vi "Analyze dIdV.vi"() -> ()   [LabVIEW 2021, in "dIdV State.lvclass"]
uses:
  dIdV State/dIdV State.lvclass
  Controls/PCS Config.ctl
  Parameters.ctl
  dIdV State/dIdV State.lvclass/dIdV State.ctl
  <vilib>/Utility/config.llb/NI_LVConfig.lvlib
  <vilib>/Utility/TDMS File Viewer/NI_TDMS File Viewer.lvlib
panel:
  in  "Array - String":string[](array[string])
  in  "Input onfiguration":T1={"File Path"=path "U:/My Documents/Projects/Eremets/NV/IV/Data/August_2022/080922/m008_080922.tdms", "from scan..."=0, "...to scan"=4, "Resistance in series"=25.65079365079365, "Correct conductance "=TRUE, "Model parameters"={"Delta"=0.025, "Gama"=0.0, "Z"=0.0, "P"=0.0, "T"=1.0, "Integration range"=2.0, "Resolution"=0.0001}, "Scale"=0.5473251028806585, "Offset"=0.0, "Other channels"=[]} {"Offset" scale=0.0..1.0; "Scale" scale=0.0..1.0; "Model parameters"."Resolution" format="%#_6peV"; "Model parameters"."Integration range" format="%#_6peV"; "Model parameters"."T" format="%#_6pK"; "Model parameters"."Delta" step=0.001 format="%#_6peV"; "Model parameters"."Gama" step=0.001 format="%#_6peV"; "Resistance in series" scale=75.0..85.0}
  in  "Tab Control":enum32{"Input", "Model", "Evaluations"}(tab)
  in  "View Button":bool
  out "Scans in file":i32
  out "All scans":cluster{dbl[], dbl[]}[](graph)
  in  "Open Button":bool
  out "Other values":string[](array[string])
  out "BTK model":cluster{dbl[], dbl[]}[](graph)
  out "V-I":cluster{"I":dbl[], dbl[]}[](graph)
  in  "Model Button":bool
  out "BSC Delta T":dbl=0.003040195174884819 format="%#_6peV"
  out "BSC Delta 0":dbl=0.003040195174884819 format="%#_6peV"
  in  "Physical quantities":T3={"Tc"=20.0, "T"=20.0, "Tc-> Delta factor"=1.764, "Hc2 at T"=20.0, "H"=20.0} {"H" format="%#_6pT"; "Hc2 at T" format="%#_6pT"; "Tc-> Delta factor" format="%#_6p"; "T" format="%#_6pK"; "Tc" format="%#_6pK"}
  out "BSC Delta T H":dbl=0.003040195174884819 format="%#_6peV"
  in  "Write cfg":bool
  in  "Read cfg":bool
  in  "Process Stop Button":bool
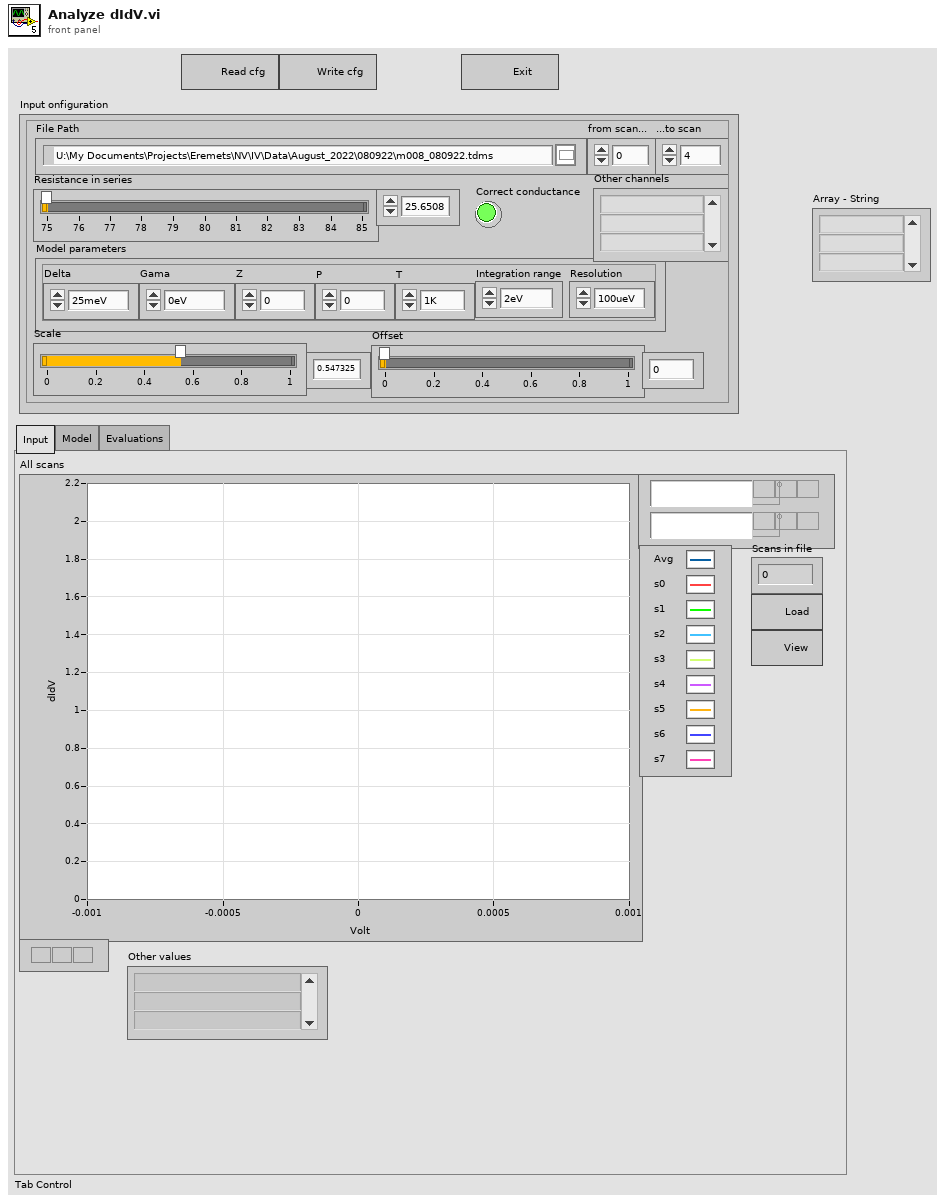
[diagram p1: front panel]
types:
  T1 = typedef "PCS Config.ctl" = cluster{"File Path":path, "from scan...":i32, "...to scan":i32, "Resistance in series":dbl, "Correct conductance ":bool, "Model parameters":T2, "Scale":dbl, "Offset":dbl, "Other channels":string[]}
  T2 = typedef "Parameters.ctl" = cluster{"Delta":dbl, "Gama":dbl, "Z":dbl, "P":dbl, "T":dbl, "Integration range":dbl, "Resolution":dbl}
  T3 = cluster{"Tc":dbl, "T":dbl, "Tc-> Delta factor":dbl, "Hc2 at T":dbl, "H":dbl}
  T4 = enum8{"Enabled", "Disabled", "Disabled and Grayed Out"}
  T5 = typedef "NI_LVConfig.lvlib/Config Data RefNum.ctl" = refnum<k1>
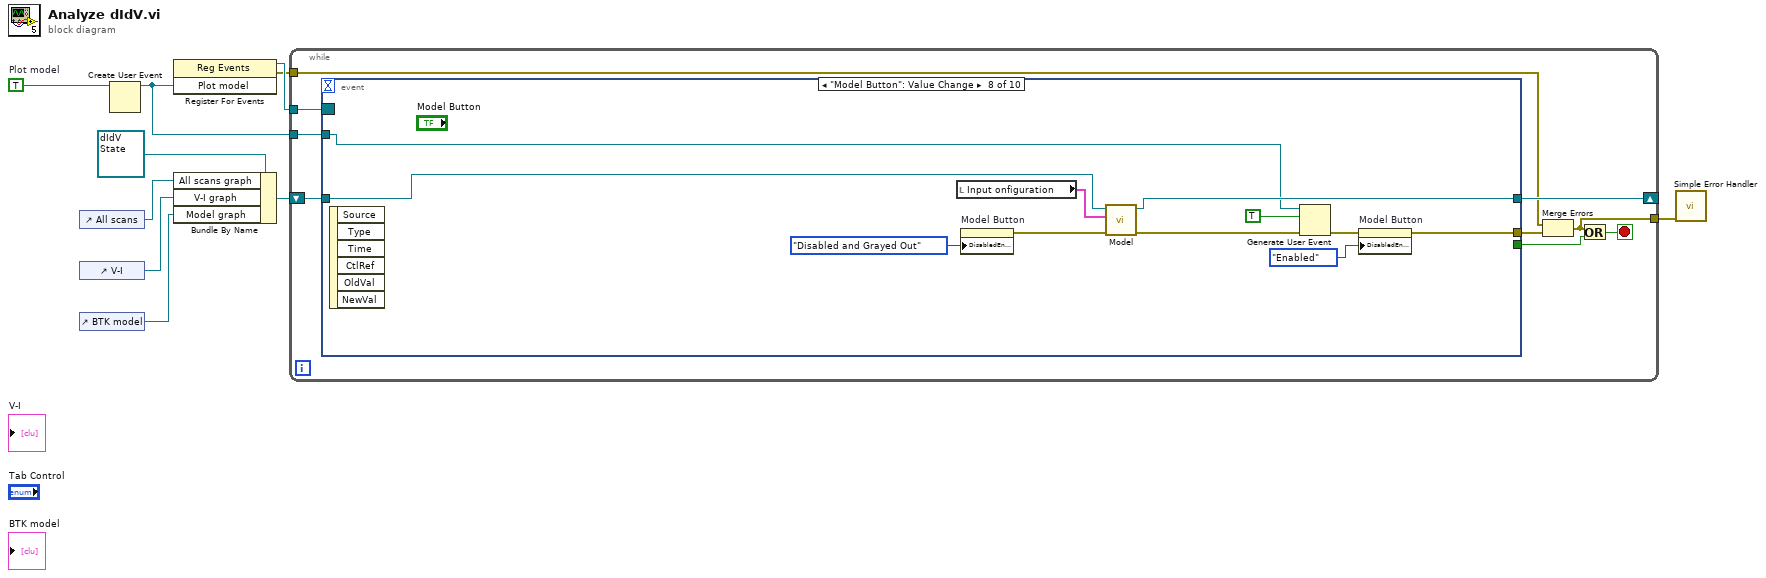
[diagram p0: block diagram]
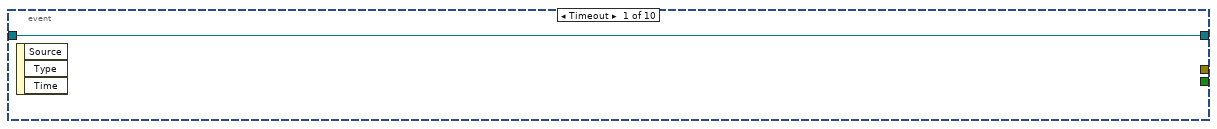
[diagram p2: hidden frame]
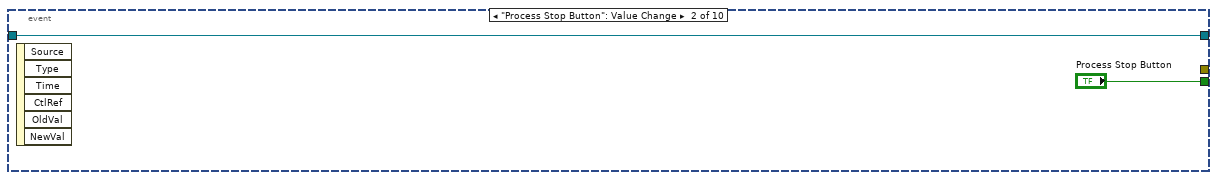
[diagram p3: hidden frame]
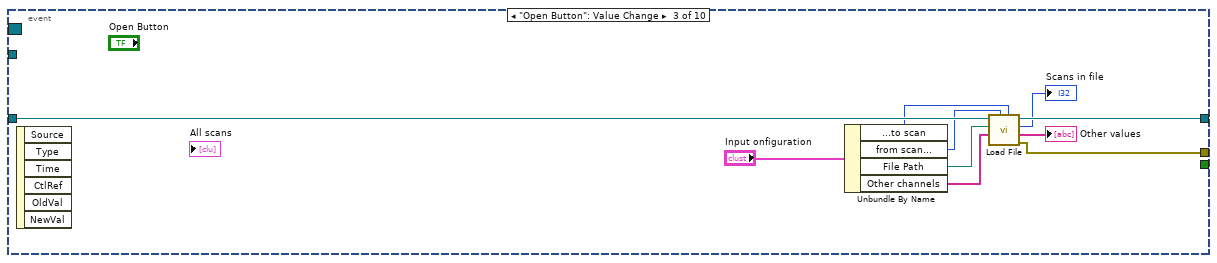
[diagram p4: hidden frame]
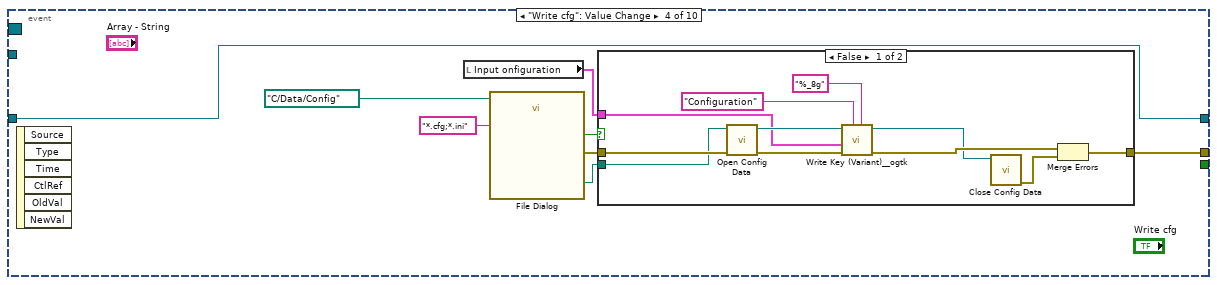
[diagram p5: hidden frame]
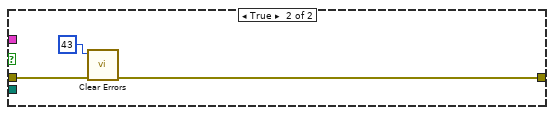
[diagram p6: hidden frame]
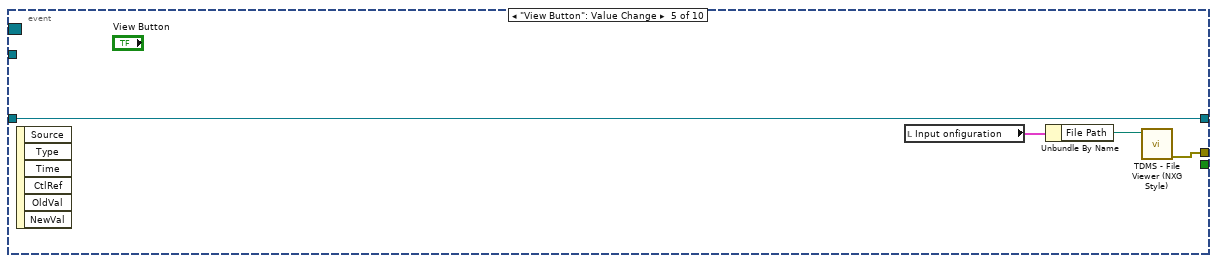
[diagram p7: hidden frame]
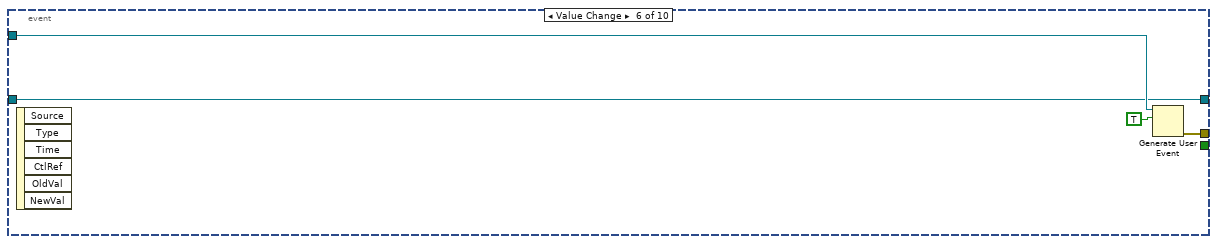
[diagram p8: hidden frame]
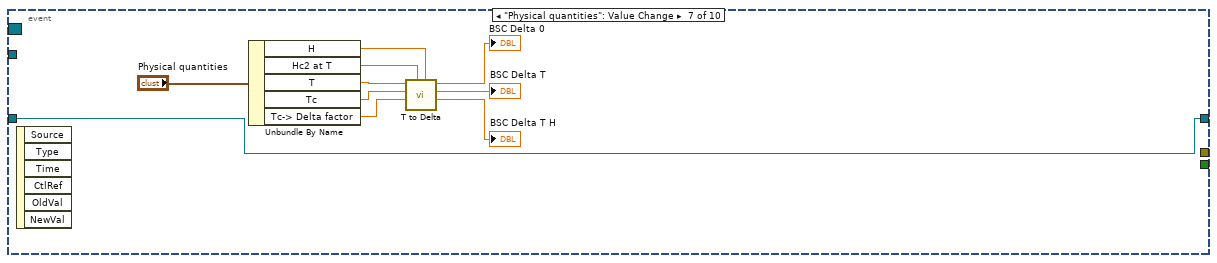
[diagram p9: hidden frame]
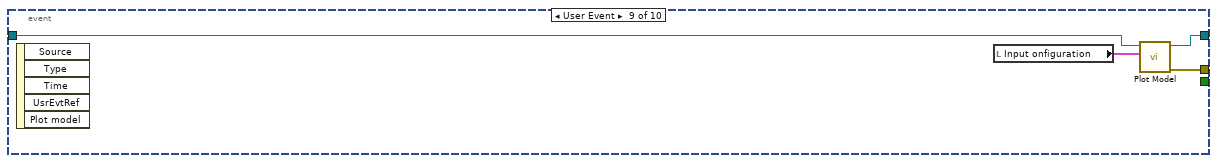
[diagram p10: hidden frame]
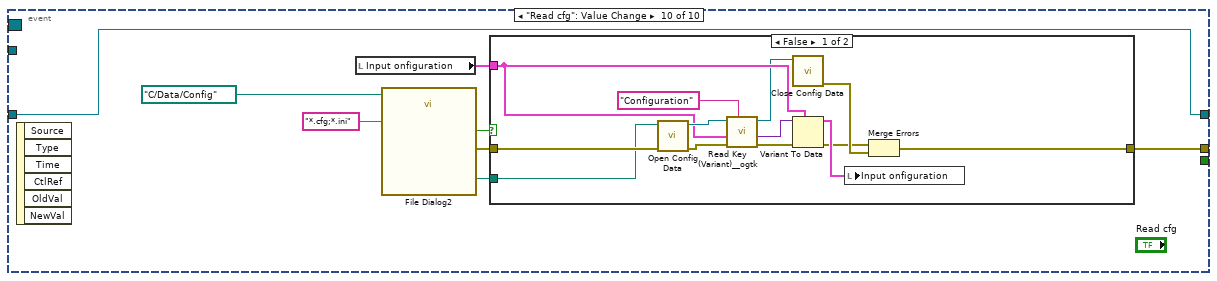
[diagram p11: hidden frame]
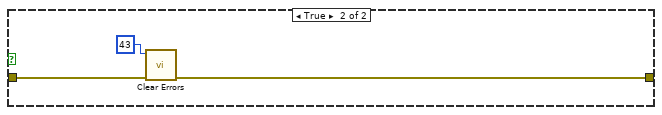
[diagram p12: hidden frame]
diagram:
  w4 = TRUE  # Plot model
  n1 = control-ref of="All scans"() -> (w8:refnum<vi>)
  n2 = control-ref of="V-I"() -> (w6:refnum<vi>)
  n3 = control-ref of="BTK model"() -> (w5:refnum<vi>)
  n4 = Create User Event(user event datatype=w4) -> (user event=w1:refnum<user-event>)  [unwired: 1 in, 1 out]
  n5 = register-events(w1) -> (reference out=w3:refnum<event-registration>, error out=w2:errorcluster)  [unwired: 2 in]
  n6 = Bundle By Name(cluster=refnum<class "dIdV State.lvclass"> refnum ("dIdV State.lvclass"), "All scans graph"=w8, "V-I graph"=w6, "Model graph"=w5) -> (w7:refnum<class "dIdV State.lvclass">)
  n7 = while {
    tunnel: [w13] -> w10
    shift-right: [w15] -> _
    shift-left: w7 -> [w16]
    tunnel: w3 -> [w14]
    tunnel: w2 -> [w12]
    tunnel: w1 -> [w11]
    stop <- w18 stop-if-true
    n8 = event shown="[7] \"Model Button\": Value Change" {
      selector: w14 -> [_ _ _ _ _ _ _ _ _ _]
      dyn-events: _ -> [_ _ _ _ _ _ _ _ _ _]
      timeout: _ -> [_ _ _ _ _ _ _ _ _ _]
      tunnel: [_ "Process Stop Button" _ _ _ _ _ _ _ _] -> w19
      tunnel: [_ _ w30 w36 w55 w61 _ w74 w85 w91] -> w17
      tunnel: w16 -> [w20 w21 w32 w35 w58 w59 w63 w83 w87 w90]
      tunnel: [w20 w21 w31 w35 w58 w59 w63 w82 w86 w90] -> w15
      tunnel: w11 -> [_ _ _ _ _ w62 _ w79 _ _]
      event Timeout {
        n9 = event-data() -> ()  [unwired: 1 in, 3 out]
      }
      event "Process Stop Button": Value Change {
        n10 = event-data() -> ()  [unwired: 1 in, 6 out]
      }
      event "Open Button": Value Change {
        n11 = event-data() -> ()  [unwired: 1 in, 6 out]
        n12 = Unbundle By Name("Input onfiguration") -> ("...to scan"=w27:i32, "from scan..."=w26:i32, "File Path"=w25:path, "Other channels"=w23:string[])
        n13 = call-dynamic "Load File.vi"("...to scan"=w27, "from scan..."=w26, "Other channels"=w23, "File Path"=w25, "dIdV State in"=w32) -> ("error out"=w30:errorcluster, "Other values"=→"Other values":string[], "Number of scans"=→"Scans in file":i32, "dIdV State out"=w31:refnum<class "dIdV State.lvclass">)  [unwired: 3 in]
      }
      event "Write cfg": Value Change {
        n14 = event-data() -> ()  [unwired: 1 in, 6 out]
        n15 = local read "Input onfiguration"() -> (w34:T1)
        n16 = call "File Dialog"("start path"=path "C:/Data/Config", "pattern (all files)"="*.cfg;*.ini") -> ("selected path"=w39:path, "cancelled"=w40:bool, "error out"=w37:errorcluster)  [unwired: 10 in, 1 out]
        n17 = case shown="False" w40 {
          tunnel: w39 -> [w44 _]
          tunnel: w37 -> [w45 w54]
          tunnel: [w42 w53] -> w36
          tunnel: w34 -> [w43 _]
          frame False {
            n18 = call <vilib>:"Open Config Data.vi"("error in (no error)"=w45, "configuration file path"=w44) -> ("error out"=w47:errorcluster, "refnum"=w46:T5)  [unwired: 7 in, 1 out]
            n19 = call <userlib>:"Write Key (Variant)__ogtk.vi"("float number format"="%_8g", "section"="Configuration", "error in (no error)"=w47, "key-value"=w43, "refnum"=w46) -> ("error out"=w49:errorcluster, "refnum out"=w48:T5)  [unwired: 5 in]
            n20 = call <vilib>:"Close Config Data.vi"("refnum"=w48) -> ("error out"=w50:errorcluster)  [unwired: 9 in, 1 out]
            n21 = Merge Errors(w49, w50) -> (w42:errorcluster)
          }
          frame True {
            n22 = call <vilib>:"Clear Errors.vi"("error in (no error)"=w54, "specific error code to clear (0: all)"=43) -> ("error out"=w53:errorcluster)  [unwired: 4 in, 1 out]
          }
        }
      }
      event "View Button": Value Change {
        n23 = event-data() -> ()  [unwired: 1 in, 6 out]
        n24 = local read "Input onfiguration"() -> (w57:T1)
        n25 = Unbundle By Name(w57) -> ("File Path"=w56:path)
        n26 = call <vilib>:"TDMS - File Viewer (NXG Style).vi"("file in"=w56) -> ("error out"=w55:errorcluster)  [unwired: 9 in, 1 out]
      }
      event Value Change {
        n27 = event-data() -> ()  [unwired: 1 in, 6 out]
        n28 = Generate User Event(user event=w62, event data cluster=TRUE ("event data")) -> (error out=w61:errorcluster)  [unwired: 2 in, 1 out]
      }
      event "Physical quantities": Value Change {
        n29 = event-data() -> ()  [unwired: 1 in, 6 out]
        n30 = Unbundle By Name("Physical quantities") -> ("H"=w68:dbl, "Hc2 at T"=w67:dbl, "T"=w71:dbl, "Tc"=w70:dbl, "Tc-> Delta factor"=w69:dbl)
        n31 = call "T to Delta.vi"("H"=w68, "Hc2 at T"=w67, "Delta Tc factor"=w69, "Tc"=w70, "T"=w71) -> ("BSC Delta T H"=→"BSC Delta T H":dbl, "BSC Delta T"=→"BSC Delta T":dbl, "BSC Delta 0"=→"BSC Delta 0":dbl)  [unwired: 4 in]
      }
      event "Model Button": Value Change {
        n32 = event-data() -> ()  [unwired: 1 in, 6 out]
        n33 = local read "Input onfiguration"() -> (w81:T1)
        n34 = property on="Model Button" class="Bool"("DisabledEnum"=T4."Disabled and Grayed Out" ("Disabled")) -> (error out=w76:errorcluster)  [unwired: 2 in, 1 out]
        n35 = call-dynamic "Model.vi"("error in (no error)"=w76, "Input onfiguration"=w81, "dIdV State in"=w83) -> ("error out"=w80:errorcluster, "dIdV State out"=w82:refnum<class "dIdV State.lvclass">)  [unwired: 7 in]
        n36 = Generate User Event(user event=w79, event data cluster=TRUE ("event data"), error in=w80) -> (error out=w75:errorcluster)  [unwired: 1 in, 1 out]
        n37 = property on="Model Button" class="Bool"(error in=w75, "DisabledEnum"=T4."Enabled" ("Disabled")) -> (error out=w74:errorcluster)  [unwired: 1 in, 1 out]
      }
      event User Event {
        n38 = event-data() -> ()  [unwired: 1 in, 5 out]
        n39 = local read "Input onfiguration"() -> (w84:T1)
        n40 = call-dynamic "Plot Model.vi"("Input onfiguration"=w84, "dIdV State in"=w87) -> ("error out"=w85:errorcluster, "dIdV State out"=w86:refnum<class "dIdV State.lvclass">)  [unwired: 8 in]
      }
      event "Read cfg": Value Change {
        n41 = event-data() -> ()  [unwired: 1 in, 6 out]
        n42 = local read "Input onfiguration"() -> (w89:T1)
        n43 = call "File Dialog2"("start path"=path "C:/Data/Config", "pattern (all files)"="*.cfg;*.ini") -> ("selected path"=w94:path, "cancelled"=w95:bool, "error out"=w92:errorcluster)  [unwired: 10 in, 1 out]
        n44 = case shown="False" w95 {
          tunnel: w94 -> [w106 _]
          tunnel: w92 -> [w107 w111]
          tunnel: [w105 w110] -> w91
          tunnel: w89 -> [w101 _]
          frame False {
            n45 = call <vilib>:"Open Config Data.vi"("error in (no error)"=w107, "configuration file path"=w106) -> ("error out"=w98:errorcluster, "refnum"=w104:T5)  [unwired: 7 in, 1 out]
            n46 = call <userlib>:"Read Key (Variant)__ogtk.vi"("section"="Configuration", "error in (no error)"=w98, "type"=w101, "refnum"=w104) -> ("error out"=w103:errorcluster, "key-value"=w102:variant, "refnum out"=w99:T5)  [unwired: 4 in, 1 out]
            n47 = call <vilib>:"Close Config Data.vi"("refnum"=w99) -> ("error out"=w108:errorcluster)  [unwired: 9 in, 1 out]
            n48 = Variant To Data(error in=w103, type=w101, Variant=w102) -> (data=w100:T1, error out=w97:errorcluster)
            n49 = local write "Input onfiguration"(w100) -> ()
            n50 = Merge Errors(w97, w108) -> (w105:errorcluster)
          }
          frame True {
            n51 = call <vilib>:"Clear Errors.vi"("error in (no error)"=w111, "specific error code to clear (0: all)"=43) -> ("error out"=w110:errorcluster)  [unwired: 4 in, 1 out]
          }
        }
      }
    }
    n52 = Merge Errors(w12, w17) -> (w13:errorcluster)
    n53 = Or(x=w13, y=w19) -> (x .or. y?=w18:bool)
  }
  n54 = call <vilib>:"Simple Error Handler.vi"("error in (no error)"=w10) -> ()  [unwired: 4 in, 5 out]
